vi "TimeStamp to Excel.vi"(1 "Time Stamp":timestamp) -> (0 "XL Time":dbl)   [LabVIEW 2020]
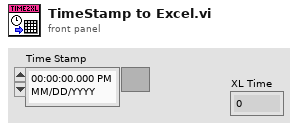
[diagram p1: front panel]
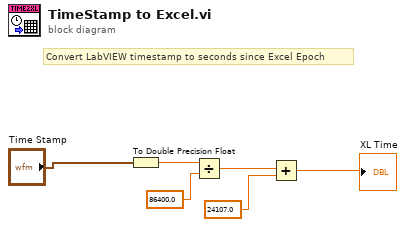
[diagram p0: block diagram]
diagram:
  # "Convert LabVIEW timestamp to seconds since Excel Epoch"
  n1 = To Double Precision Float(number="Time Stamp") -> (double precision float=w5:dbl)
  n2 = Divide(x=w5, y=86400.0) -> (x/y=w4:dbl)
  n3 = Add(x=w4, y=24107.0) -> (x+y=→"XL Time":dbl)
